vi "vi server run VI.vi"   [LabVIEW 2013, in "NISE Tools VI Server.lvlib"]
doc: "Runs a VI using the run VI method, providing it with any input parameters. This polymorph accepts either a path or a refnum."
uses:
  NISE Tools VI Server.lvlib
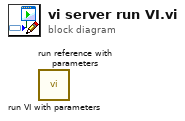
[diagram p0: block diagram]
diagram:
  n1 = call "run VI with parameters.vi"() -> ()  [unwired: 11 in, 1 out]
  n2 = call "run reference with parameters.vi"() -> ()  [unwired: 11 in, 1 out]
